vi "Actor Core.vi"(8 "error in":errorcluster, 11 "Abstract Display in":refnum<class "Abstract Display.lvclass">) -> (0 "error out":errorcluster, 3 "Actor out":refnum<class "Actor.lvclass">)   [LabVIEW 2014, in "Display Panel.lvlib" / "Abstract Display.lvclass"]
doc: "(<B>Filename</B>: Actor Framework.lvlib:Actor.lvclass:Actor Core.vi)\n\nReceives messages to the actor, reacts to them, and initiates any error handling that may shut the actor down.\n\nDescendant classes may override this VI to append parallel tasks for the actor to complete while it handles messages. Overrides use the Call Parent Method node."
uses:
  Abstract Display.lvclass
  <vilib>/ActorFramework/Actor/Actor.lvclass
  State.ctl
  Abstract Display.lvclass/Abstract Display.ctl
  <vilib>/MGI/Monitored Actor/Actor/Monitored Actor.lvclass
  Display Panel.lvlib
panel:
  out "resulting string":string
  out "Elapsed Time (s)":dbl
  out "i":i32
  in  "Value":T1=enum."Warming"
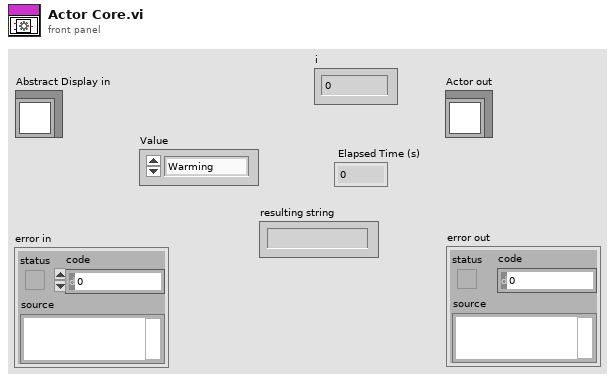
[diagram p1: front panel]
types:
  T1 = typedef "Display Panel.lvlib/Abstract Display.lvclass/State.ctl" = enum16{"Done", "Warming", "Measuring"}
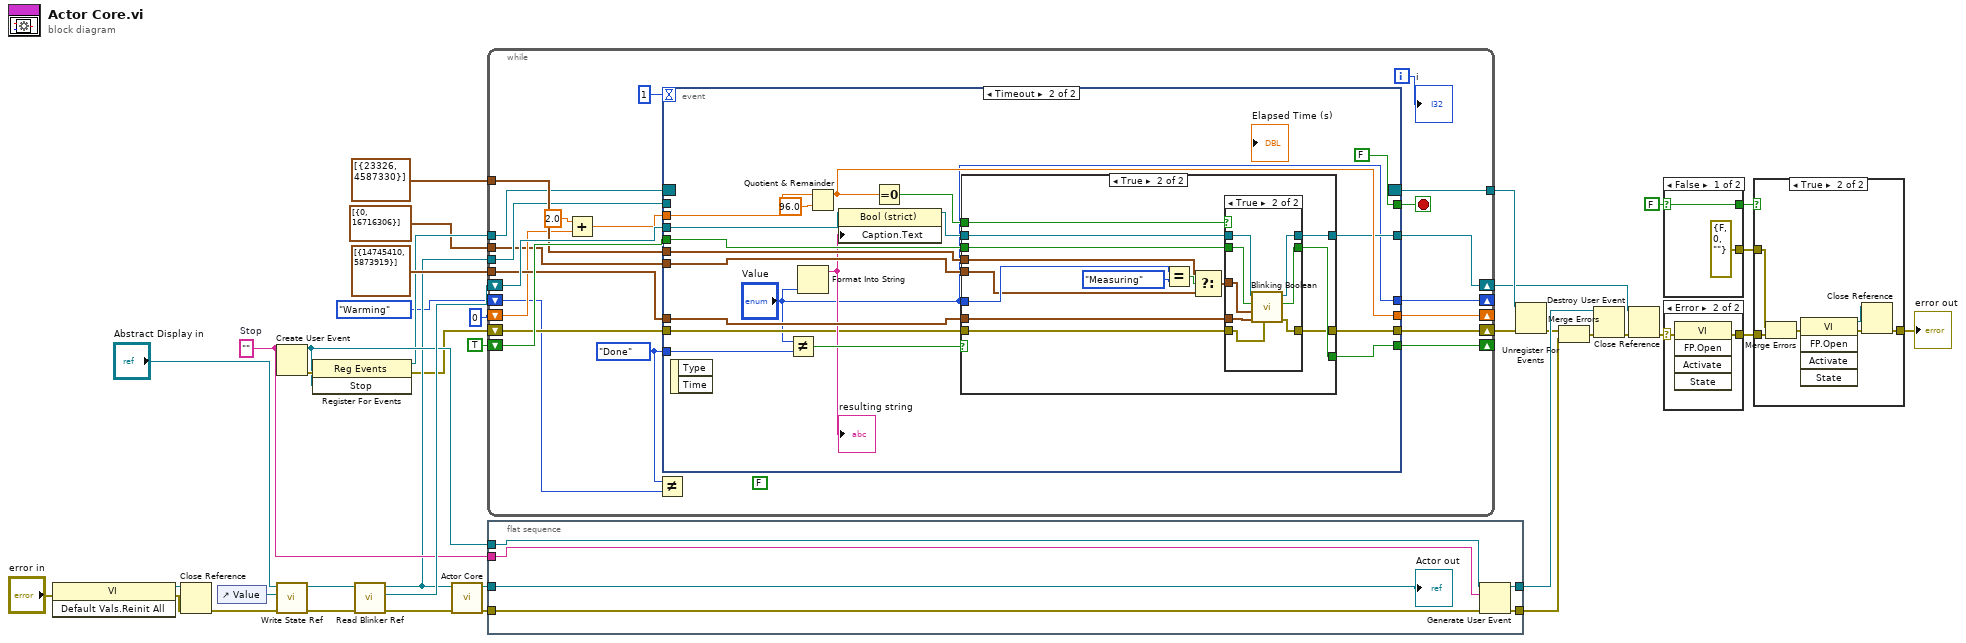
[diagram p0: block diagram]
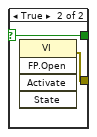
[diagram p4: hidden frame]
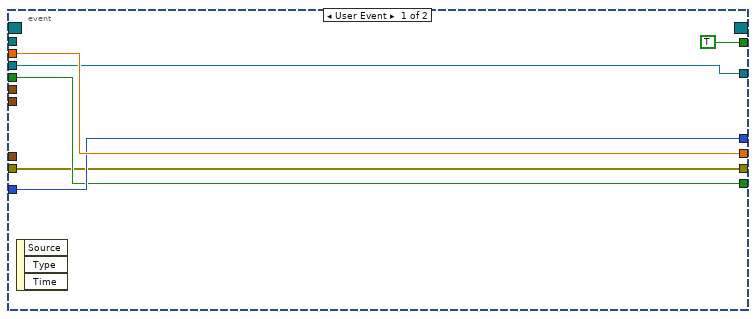
[diagram p5: hidden frame]
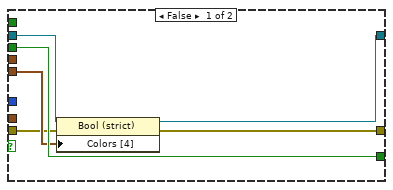
[diagram p6: hidden frame]
diagram:
  w27 = ""  # Stop
  n1 = invoke class="VI" method="Default Vals.Reinit All"(error in="error in") -> (reference out=w12:refnum<vi>, error out=w11:errorcluster)  [unwired: 2 in, 1 out]
  n2 = Close Reference(reference=w12, error in (no error)=w11) -> (error out=w10:errorcluster)
  n3 = control-ref of="Value"() -> (w17:refnum<vi>)
  n4 = Create User Event(user event datatype=w27) -> (user event=w30:refnum<user-event>, error out=w31:errorcluster)  [unwired: 1 in]
  n5 = call "Write State Ref.vi"("error in (no error)"=w10, "State Ref"=w17, "Abstract Display in"="Abstract Display in") -> ("error out"=w18:errorcluster, "Abstract Display out"=w19:refnum<class "Abstract Display.lvclass">)  [unwired: 7 in]
  n6 = register-events(error in=w31, w30) -> (reference out=w29:refnum<event-registration>, error out=w9:errorcluster)  [unwired: 1 in]
  n7 = call "Read Blinker Ref.vi"("error in (no error)"=w18, "Abstract Display in"=w19) -> ("error out"=w26:errorcluster, "Blinker Ref"=w36:refnum<vi>, "Abstract Display out"=w25:refnum<class "Abstract Display.lvclass">)  [unwired: 7 in]
  n8 = call-parent "Actor Core.vi"("error in"=w26, "Actor in"=w25) -> ("error out"=w38:errorcluster, "Actor out"=w37:refnum<class "Actor.lvclass">)  [unwired: 8 in]
  n9 = while {
    shift-right: [w58] -> _
    shift-left: TRUE -> [w59]
    tunnel: cluster{u32, u32}[] [{23326, 4587330}] ("Color 2 (Background, Foreground)") -> [w57]
    tunnel: cluster{u32, u32}[] [{14745410, 5873919}] ("Colors [4]") -> [w56]
    tunnel: w29 -> [w55]
    tunnel: [w54] -> w28
    tunnel: w25 -> [w53]
    shift-right: [w50] -> _
    shift-left: 0 -> [w52]
    tunnel: cluster{u32, u32}[] [{0, 16716306}] ("Colors [4]") -> [w49]
    shift-right: [w48] -> _
    shift-left: State."Warming" ("y") -> [w41]
    shift-right: [w47] -> w21
    shift-left: w9 -> [w46]
    shift-right: [w39] -> w6
    shift-left: w36 -> [w60]
    i -> [w43]
    stop <- w44 stop-if-true
    (unwired) FALSE
    w42 = State."Done" ("y")
    n10 = Add(x=2.0, y=w52) -> (x+y=w51:dbl)
    n11 = Not Equal?(x=w42, y=w41) -> ()  [unwired: 1 out]
    n12 = event shown="[1] Timeout" {
      selector: w55 -> [_ _]
      dyn-events: [_ _] -> w54
      timeout: 1 -> [_ _]
      tunnel: w60 -> [w61 w75]
      tunnel: w59 -> [w63 w84]
      tunnel: [w63 w83] -> w58
      tunnel: w57 -> [_ w82]
      tunnel: w56 -> [_ w81]
      tunnel: [TRUE FALSE] -> w44
      tunnel: w53 -> [_ _]
      tunnel: w51 -> [w65 w80]
      tunnel: [w65 w79] -> w50
      tunnel: w49 -> [_ w78]
      tunnel: [w64 "Value"] -> w48
      tunnel: [w62 w72] -> w47
      tunnel: w46 -> [w62 w71]
      tunnel: w42 -> [w64 w70]
      tunnel: [w61 w68] -> w39
      event User Event {
        n13 = event-data() -> ()  [unwired: 1 in, 3 out]
      }
      event Timeout {
        n14 = event-data() -> ()  [unwired: 1 in, 2 out]
        n15 = Not Equal?(x="Value", y=w70) -> (x != y?=w77:bool)
        n16 = Format Into String("Value") -> (resulting string=w73:string)  [unwired: 3 in, 1 out]
        "resulting string" <- w73
        n17 = Quotient & Remainder(x=w80, y=96.0) -> (x-y*floor(x/y)=w79:dbl)  [unwired: 1 out]
        n18 = property class="Bool (strict)"(reference=w75, "Caption.Text"=w73) -> (reference out=w74:refnum<vi>)  [unwired: 1 in, 1 out]
        n19 = Equal To 0?(x=w79) -> (x = 0?=w76:bool)
        n20 = case shown="True" w77 {
          tunnel: w74 -> [w90 w105]
          tunnel: w84 -> [w91 w104]
          tunnel: [w91 w103] -> w83
          tunnel: w82 -> [_ w98]
          tunnel: w81 -> [_ w102]
          tunnel: w78 -> [w89 w96]
          tunnel: "Value" -> [_ w100]
          tunnel: w76 -> [_ w95]
          tunnel: [w88 w93] -> w72
          tunnel: w71 -> [w86 w94]
          tunnel: [w87 w92] -> w68
          frame False {
            n21 = property class="Bool (strict)"(reference=w90, error in=w86, "Colors [4]"=w89) -> (reference out=w87:refnum<vi>, error out=w88:errorcluster)
          }
          frame True {
            n22 = Equal?(x=w100, y=State."Measuring") -> (x = y?=w101:bool)
            n23 = Select(t=w98, s=w101, f=w96) -> (s? t:f=w97:cluster{u32, u32}[])
            n24 = case shown="True" w95 {
              tunnel: w105 -> [w106 w116]
              tunnel: w104 -> [w108 w115]
              tunnel: [w108 w114] -> w103
              tunnel: w102 -> [_ w113]
              tunnel: w97 -> [_ w112]
              tunnel: w94 -> [w107 w111]
              tunnel: [w107 w110] -> w93
              tunnel: [w106 w109] -> w92
              frame False {
              }
              frame True {
                n25 = call "Blinking Boolean.vi"("Error In"=w111, "Color 2 (Background, Foreground)"=w113, "Color 1 (Background, Foreground)"=w112, "Shift in"=w115, "Bool Refnum"=w116) -> ("Error Out"=w110:errorcluster, "Shift out"=w114:bool, "reference out"=w109:refnum<vi>)  [unwired: 4 in]
              }
            }
          }
        }
      }
    }
    "i" <- w43
  }
  n26 = flat-sequence {
    tunnel: w38 -> [w119]
    tunnel: w37 -> [w122]
    tunnel: [w121] -> w32
    tunnel: [w120] -> w14
    tunnel: w30 -> [w118]
    tunnel: w27 -> [w117]
    frame #0 {
      n27 = Generate User Event(user event=w118, event data cluster=w117, error in=w119) -> (user event out=w121:refnum<user-event>, error out=w120:errorcluster)  [unwired: 1 in]
      "Actor out" <- w122
    }
  }
  n28 = Unregister For Events(event registration refnum=w28, error in=w21) -> (error out=w15:errorcluster)
  n29 = Merge Errors(w15, w14) -> (w13:errorcluster)
  n30 = Destroy User Event(user event=w32, error in=w13) -> (error out=w8:errorcluster)
  n31 = Close Reference(reference=w6, error in (no error)=w8) -> (error out=w7:errorcluster)
  n32 = case shown="False" FALSE {
    selector: FALSE -> [w124 w126]
    tunnel: [w124 w126] -> w4
    tunnel: [errorcluster {"status"=FALSE, "code"=0, "source"=""} ("error out") w125] -> w2
    frame False {
    }
    frame True {
      n33 = invoke class="VI" method="FP.Open"() -> (error out=w125:errorcluster)  [unwired: 5 in, 4 out]
    }
  }
  n34 = case shown="Error" w7 {
    selector: w7 -> [w127 w129]
    tunnel: [w127 w128] -> w1
    frame No Error {
    }
    frame Error {
      n35 = invoke class="VI" method="FP.Open"(error in=w129) -> (error out=w128:errorcluster)  [unwired: 4 in, 4 out]
    }
  }
  n36 = case shown="True" w4 {
    tunnel: [w130 w134] -> w3
    tunnel: w2 -> [w130 w133]
    tunnel: w1 -> [_ w132]
    frame False {
    }
    frame True {
      n37 = Merge Errors(w133, w132) -> (w131:errorcluster)
      n38 = invoke class="VI" method="FP.Open"(error in=w131) -> (reference out=w135:refnum<vi>, error out=w136:errorcluster)  [unwired: 4 in, 3 out]
      n39 = Close Reference(reference=w135, error in (no error)=w136) -> (error out=w134:errorcluster)
    }
  }
  "error out" <- w3
